vi "subthing.vi"(10 "Cluster":T1={"Drag"=0.0, "gravity(in/s^2)"=-386.09, "Minimum Goal Height(in)"=85.0, "Ideal Height(in)"=0.0, "Maximum Goal Height(in)"=109.0, "xspeed"=0.0, "yspeed"=0.0, "xpos"=0.0, "ypos"=0.0, "Frametime"=0.0}) -> (2 "output cluster":T1)   [LabVIEW 2015]
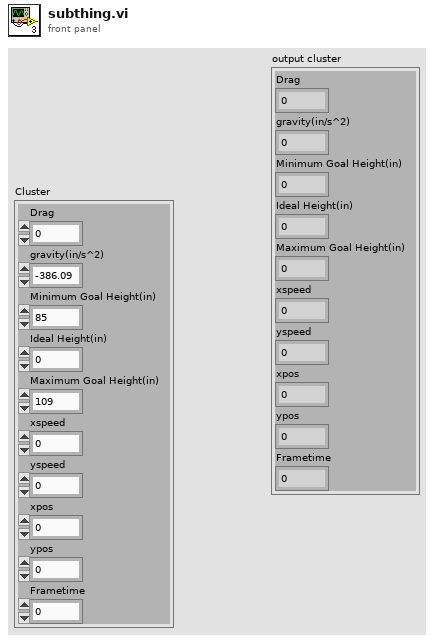
[diagram p1: front panel]
types:
  T1 = cluster{"Drag":dbl, "gravity(in/s^2)":dbl, "Minimum Goal Height(in)":dbl, "Ideal Height(in)":dbl, "Maximum Goal Height(in)":dbl, "xspeed":dbl, "yspeed":dbl, "xpos":dbl, "ypos":dbl, "Frametime":dbl}
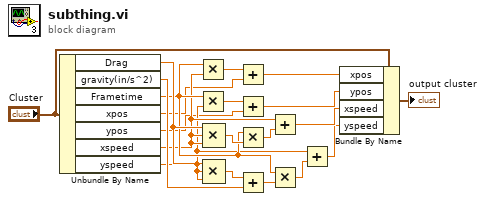
[diagram p0: block diagram]
diagram:
  n1 = Unbundle By Name("Cluster") -> ("Drag"=w12:dbl, "gravity(in/s^2)"=w13:dbl, "Frametime"=w11:dbl, "xpos"=w4:dbl, "ypos"=w2:dbl, "xspeed"=w9:dbl, "yspeed"=w3:dbl)
  n2 = Multiply(x=w11, y=w9) -> (x*y=w15:dbl)
  n3 = Multiply(x=w11, y=w3) -> (x*y=w14:dbl)
  n4 = Compound Arithmetic op=MULTIPLY(w12, w9, w9) -> (w17:dbl)
  n5 = Compound Arithmetic op=MULTIPLY(w12, w3, w3) -> (w20:dbl)
  n6 = Add(x=w15, y=w4) -> (x+y=w6:dbl)
  n7 = Add(x=w14, y=w2) -> (x+y=w7:dbl)
  n8 = Multiply(x=w11, y=w17) -> (x*y=w16:dbl)
  n9 = Add(x=w20, y=w13) -> (x+y=w19:dbl)
  n10 = Add(x=w9, y=w16) -> (x+y=w8:dbl)
  n11 = Multiply(x=w11, y=w19) -> (x*y=w18:dbl)
  n12 = Add(x=w3, y=w18) -> (x+y=w5:dbl)
  n13 = Bundle By Name(cluster="Cluster", "xpos"=w6, "ypos"=w7, "xspeed"=w8, "yspeed"=w5) -> (→"output cluster":T1)
